vi "NML_DATA_ACQ_Control_mem.vi"(1 "comments":string, 2 "NML Data Acquisition VI":string(combo)="NML Data Acquisition-New.vi", 3 "Enum":T1(ring), 4 "Trigger Column":i32, 5 "Æ Trigger":dbl=0.1) -> (0 "started":bool)   [LabVIEW 2020]
panel:
  # "Some functions not working with \nNML data acquisition-new.vi"
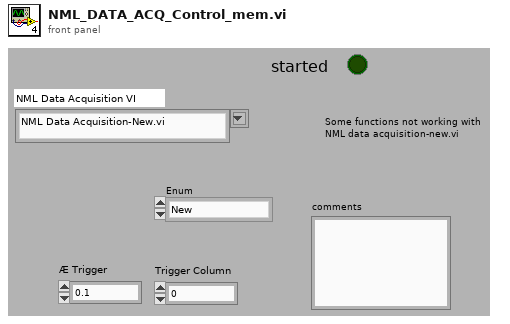
[diagram p1: front panel]
types:
  T1 = enum32{"New", "Stop", "Trigger", "Delta Trigger", "Run", "Pause", "comments", "Started?"}
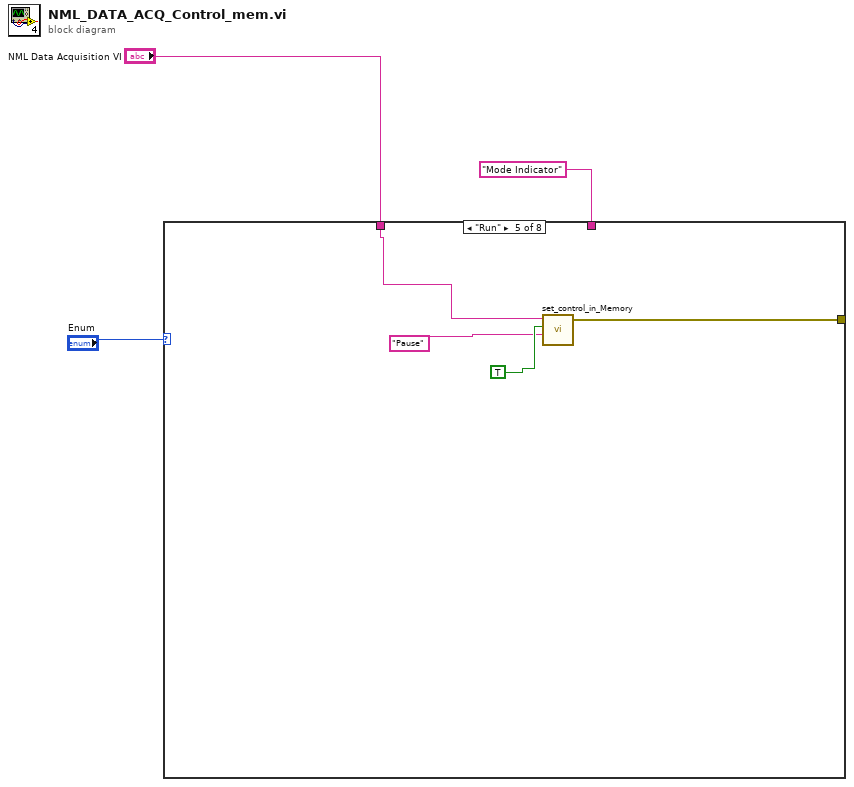
[diagram p0: block diagram]
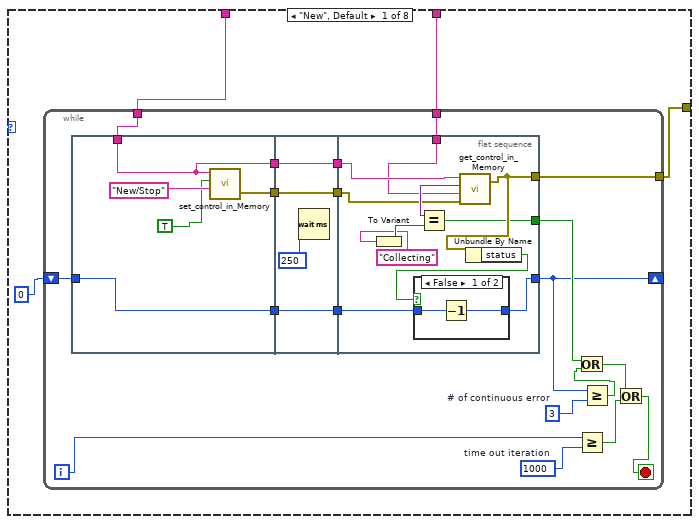
[diagram p2: hidden frame]
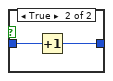
[diagram p3: hidden frame]
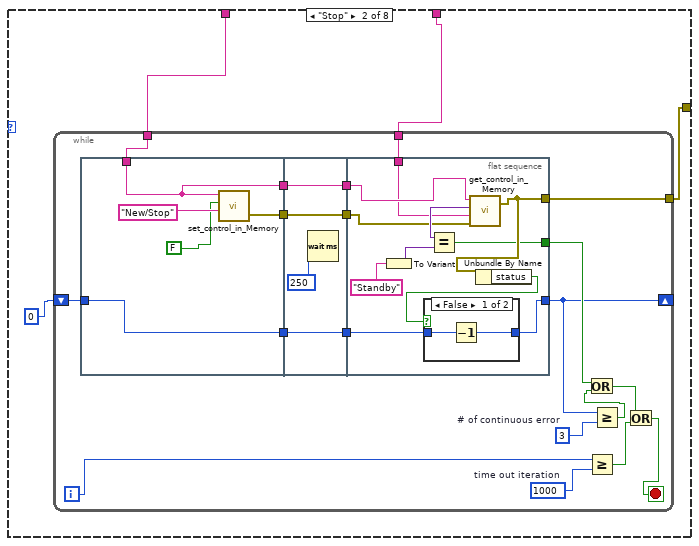
[diagram p4: hidden frame]
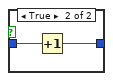
[diagram p5: hidden frame]
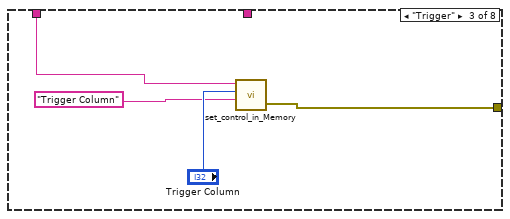
[diagram p6: hidden frame]
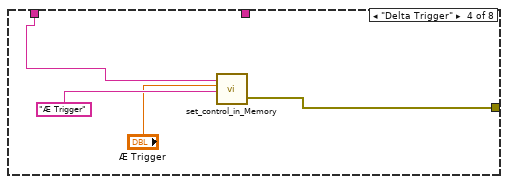
[diagram p7: hidden frame]
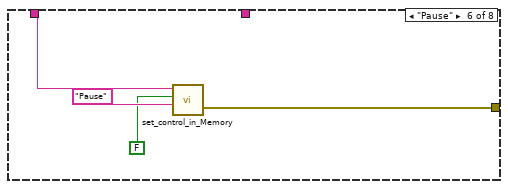
[diagram p8: hidden frame]
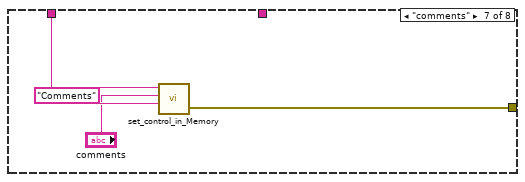
[diagram p9: hidden frame]
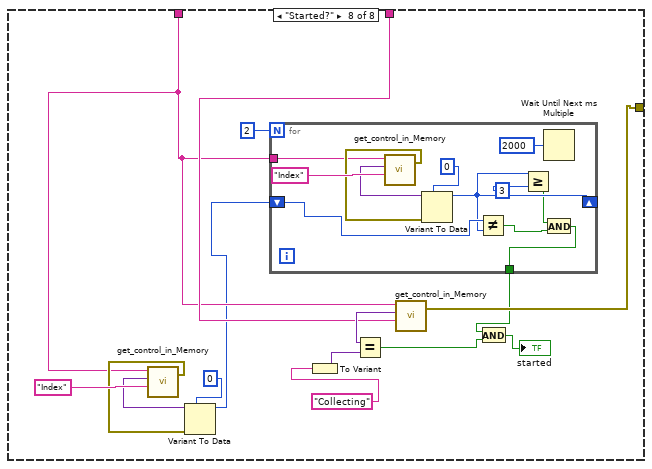
[diagram p10: hidden frame]
diagram:
  n1 = case shown="\"Run\"" "Enum" {
    tunnel: [w4 w52 w99 w103 w107 w111 w116 w120] -> _
    tunnel: "NML Data Acquisition VI" -> [w6 w51 w98 w102 w106 w110 w114 w122]
    tunnel: "Mode Indicator" ("Control Name") -> [w5 w53 _ _ _ _ _ w129]
    frame "New", Default {
      n2 = while {
        tunnel: w6 -> [w26]
        tunnel: [w25] -> w4
        shift-right: [w18] -> _
        shift-left: i16 0 -> [w20]
        tunnel: w5 -> [w8]
        i -> [w15]
        stop <- w11 stop-if-true
        w14 = 1000  # time out iteration
        w17 = i16 3  # # of continuous error
        n3 = flat-sequence {
          tunnel: w26 -> [w27]
          tunnel: [w30] -> w24
          tunnel: [w28] -> w21
          tunnel: w20 -> [w28]
          tunnel: [w27] -> w10
          tunnel: w24 -> [w35]
          tunnel: [w35] -> w23
          tunnel: [w33] -> w22
          tunnel: w21 -> [w33]
          tunnel: w10 -> [w32]
          tunnel: [w32] -> w9
          tunnel: w23 -> [w44]
          tunnel: [w43] -> w25
          tunnel: [w41] -> w18
          tunnel: w22 -> [w40]
          tunnel: [w39] -> w19
          tunnel: w9 -> [w38]
          tunnel: w8 -> [w37]
          frame #0 {
            n4 = call "set_control_in_Memory.vi"("Control Name"="New/Stop", "Value"=TRUE, "VI Name"=w27) -> ("error out 2"=w30:errorcluster)  [unwired: 2 out]
          }
          frame #1 {
            n5 = Wait (ms)(milliseconds to wait=u32 250) -> ()  [unwired: 1 out]
          }
          frame #2 {
            n6 = To Variant(anything="Collecting" ("Control Name")) -> (Variant=w46:variant)
            n7 = call "get_control_in_Memory.vi"("error in (no error)"=w44, "Control Name"=w37, "VI Name"=w38) -> ("error out 2"=w43:errorcluster, "Value"=w45:variant)  [unwired: 1 out]
            n8 = Equal?(x=w45, y=w46) -> (x = y?=w39:bool)
            n9 = Unbundle By Name(w43) -> ("status"=w42:bool)
            n10 = case shown="False" w42 {
              tunnel: [w47 w49] -> w41
              tunnel: w40 -> [w48 w50]
              frame False {
                n11 = Decrement(x=w48) -> (x-1=w47:i16)
              }
              frame True {
                n12 = Increment(x=w50) -> (x+1=w49:i16)
              }
            }
          }
        }
        n13 = Greater Or Equal?(x=w15, y=w14) -> (x >= y?=w12:bool)
        n14 = Greater Or Equal?(x=w18, y=w17) -> (x >= y?=w16:bool)
        n15 = Or(x=w19, y=w16) -> (x .or. y?=w13:bool)
        n16 = Or(x=w13, y=w12) -> (x .or. y?=w11:bool)
      }
    }
    frame "Stop" {
      n17 = while {
        tunnel: w51 -> [w73]
        tunnel: [w72] -> w52
        shift-right: [w65] -> _
        shift-left: i16 0 -> [w67]
        tunnel: w53 -> [w55]
        i -> [w62]
        stop <- w58 stop-if-true
        w61 = 1000  # time out iteration
        w64 = i16 3  # # of continuous error
        n18 = flat-sequence {
          tunnel: w73 -> [w74]
          tunnel: [w77] -> w71
          tunnel: [w75] -> w68
          tunnel: w67 -> [w75]
          tunnel: [w74] -> w57
          tunnel: w71 -> [w82]
          tunnel: [w82] -> w70
          tunnel: [w80] -> w69
          tunnel: w68 -> [w80]
          tunnel: w57 -> [w79]
          tunnel: [w79] -> w56
          tunnel: w70 -> [w91]
          tunnel: [w90] -> w72
          tunnel: [w88] -> w65
          tunnel: w69 -> [w87]
          tunnel: [w86] -> w66
          tunnel: w56 -> [w85]
          tunnel: w55 -> [w84]
          frame #0 {
            n19 = call "set_control_in_Memory.vi"("Control Name"="New/Stop", "Value"=FALSE, "VI Name"=w74) -> ("error out 2"=w77:errorcluster)  [unwired: 2 out]
          }
          frame #1 {
            n20 = Wait (ms)(milliseconds to wait=u32 250) -> ()  [unwired: 1 out]
          }
          frame #2 {
            n21 = To Variant(anything="Standby" ("Control Name")) -> (Variant=w93:variant)
            n22 = call "get_control_in_Memory.vi"("error in (no error)"=w91, "Control Name"=w84, "VI Name"=w85) -> ("error out 2"=w90:errorcluster, "Value"=w92:variant)  [unwired: 1 out]
            n23 = Equal?(x=w92, y=w93) -> (x = y?=w86:bool)
            n24 = Unbundle By Name(w90) -> ("status"=w89:bool)
            n25 = case shown="False" w89 {
              tunnel: [w94 w96] -> w88
              tunnel: w87 -> [w95 w97]
              frame False {
                n26 = Decrement(x=w95) -> (x-1=w94:i16)
              }
              frame True {
                n27 = Increment(x=w97) -> (x+1=w96:i16)
              }
            }
          }
        }
        n28 = Greater Or Equal?(x=w62, y=w61) -> (x >= y?=w59:bool)
        n29 = Greater Or Equal?(x=w65, y=w64) -> (x >= y?=w63:bool)
        n30 = Or(x=w66, y=w63) -> (x .or. y?=w60:bool)
        n31 = Or(x=w60, y=w59) -> (x .or. y?=w58:bool)
      }
    }
    frame "Trigger" {
      n32 = call "set_control_in_Memory.vi"("Control Name"="Trigger Column", "Value"="Trigger Column", "VI Name"=w98) -> ("error out 2"=w99:errorcluster)  [unwired: 2 in]
    }
    frame "Delta Trigger" {
      n33 = call "set_control_in_Memory.vi"("Control Name"="Æ Trigger", "Value"="Æ Trigger", "VI Name"=w102) -> ("error out 2"=w103:errorcluster)  [unwired: 2 in]
    }
    frame "Run" {
      n34 = call "set_control_in_Memory.vi"("Control Name"="Pause", "Value"=TRUE, "VI Name"=w106) -> ("error out 2"=w107:errorcluster)  [unwired: 2 in]
    }
    frame "Pause" {
      n35 = call "set_control_in_Memory.vi"("Control Name"="Pause", "Value"=FALSE, "VI Name"=w110) -> ("error out 2"=w111:errorcluster)  [unwired: 2 in]
    }
    frame "comments" {
      n36 = call "set_control_in_Memory.vi"("Control Name"="Comments", "Value"="comments", "VI Name"=w114) -> ("error out 2"=w116:errorcluster)  [unwired: 2 in]
    }
    frame "Started?" {
      n37 = call "get_control_in_Memory.vi"("Control Name"="Index", "VI Name"=w122) -> ("error out 2"=w123:errorcluster, "Value"=w125:variant)  [unwired: 1 in, 1 out]
      n38 = Variant To Data(error in=w123, type=0, Variant=w125) -> (data=w121:i32)  [unwired: 1 out]
      n39 = for {
        N: 2 -> [_]
        tunnel: w122 -> [w140]
        shift-right: [w138] -> _
        shift-left: w121 -> [w139]
        tunnel: [w134] -> w118
        n40 = call "get_control_in_Memory.vi"("Control Name"="Index", "VI Name"=w140) -> ("error out 2"=w141:errorcluster, "Value"=w143:variant)  [unwired: 1 in, 1 out]
        n41 = Variant To Data(error in=w141, type=0, Variant=w143) -> (data=w138:i32)  [unwired: 1 out]
        n42 = Not Equal?(x=w139, y=w138) -> (x != y?=w135:bool)
        n43 = Greater Or Equal?(x=w138, y=3) -> (x >= y?=w136:bool)
        n44 = Wait Until Next ms Multiple(millisecond multiple=u32 2000) -> ()  [unwired: 1 out]
        n45 = And(x=w136, y=w135) -> (x .and. y?=w134:bool)
      }
      n46 = To Variant(anything="Collecting" ("Control Name")) -> (Variant=w132:variant)
      n47 = call "get_control_in_Memory.vi"("Control Name"=w129, "VI Name"=w122) -> ("error out 2"=w120:errorcluster, "Value"=w131:variant)  [unwired: 1 in, 1 out]
      n48 = Equal?(x=w131, y=w132) -> (x = y?=w128:bool)
      n49 = And(x=w118, y=w128) -> (x .and. y?=→"started":bool)
    }
  }
